vi "HightRectangle.vi"(11 "yInput":i16) -> (3 "yOutput":i16)   [LabVIEW 2014]
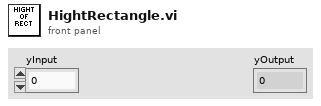
[diagram p1: front panel]
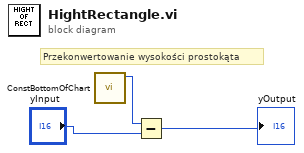
[diagram p0: block diagram]
diagram:
  # "Przekonwertowanie wysokości prostokąta"
  n1 = call "ConstBottomOfChart.vi"() -> ("bottom of rectagle"=w1:i16)  [unwired: 11 in]
  n2 = Subtract(x=w1, y="yInput") -> (x-y=→"yOutput":i16)
